vi "MOKO_Graph_main_stm.vi"(8 "error in":errorcluster, 9 "StateMachineSteps":T1[](array[typedef]), 10 "FNs":enum16{"Back", "Front", "Replace"}(ring), 11 "queue in":refnum<queue>) -> (0 "error out":errorcluster, 3 "queue out":refnum<queue>)   [LabVIEW 2018]
uses:
  MOKO_Graph_main_STM.ctl
  MOKO_Graph_main_ITEM.ctl
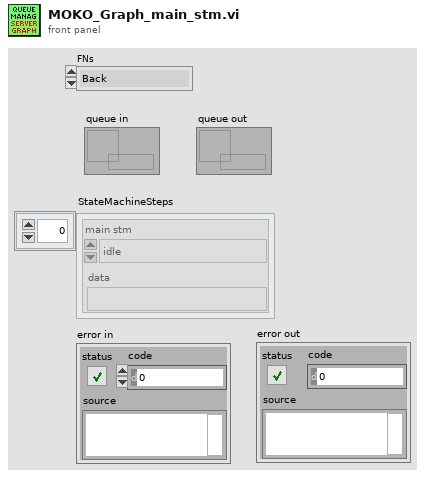
[diagram p1: front panel]
types:
  T1 = typedef "MOKO_Graph_main_STM.ctl" = cluster{"main stm":T2, "data":string}
  T2 = typedef "MOKO_Graph_main_ITEM.ctl" = enum16{"idle", "Graph read", "Graph write"}
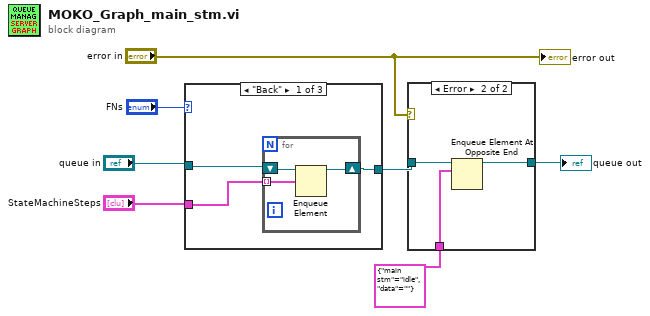
[diagram p0: block diagram]
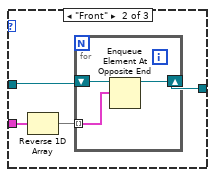
[diagram p3: hidden frame]
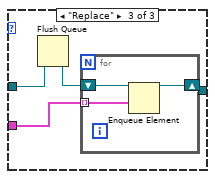
[diagram p4: hidden frame]
diagram:
  n1 = case shown="\"Back\"" "FNs" {
    tunnel: "StateMachineSteps" -> [w8 w14 w22]
    tunnel: "queue in" -> [w10 w16 w24]
    tunnel: [w9 w15 w21] -> w6
    frame "Back" {
      n2 = for {
        shift-right: [w12] -> w9
        shift-left: w10 -> [w13]
        tunnel: w8 -> [w11] mode=indexing
        n3 = Enqueue Element(queue=w13, element=w11) -> (queue out=w12:refnum<queue>)  [unwired: 2 in, 2 out]
      }
    }
    frame "Front" {
      n4 = Reverse 1D Array(array=w14) -> (reversed array=w17:T1[])
      n5 = for {
        tunnel: w17 -> [w19] mode=indexing
        shift-right: [w18] -> w15
        shift-left: w16 -> [w20]
        n6 = Enqueue Element At Opposite End(queue=w20, element=w19) -> (queue out=w18:refnum<queue>)  [unwired: 2 in, 2 out]
      }
    }
    frame "Replace" {
      n7 = Flush Queue(queue=w24) -> (queue out=w23:refnum<queue>)  [unwired: 1 in, 2 out]
      n8 = for {
        tunnel: w22 -> [w26] mode=indexing
        shift-right: [w25] -> w21
        shift-left: w23 -> [w27]
        n9 = Enqueue Element(queue=w27, element=w26) -> (queue out=w25:refnum<queue>)  [unwired: 2 in, 2 out]
      }
    }
  }
  n10 = case shown="Error" "error in" {
    tunnel: w6 -> [w28 w31]
    tunnel: [w28 w30] -> w3
    tunnel: T1 {"main stm"=enum."idle", "data"=""} ("element") -> [_ w29]
    frame No Error {
    }
    frame Error {
      n11 = Enqueue Element At Opposite End(queue=w31, element=w29) -> (queue out=w30:refnum<queue>)  [unwired: 2 in, 2 out]
    }
  }
  "queue out" <- w3
  "error out" <- "error in"
